vi "ModifyExistingBins.vi"(8 "error in (no error)":errorcluster, 11 "Node Ptr":u64 format="%.0x") -> (0 "error out":errorcluster)   [LabVIEW 2012, in "Histogram Custom Device.lvlib"]
uses:
  Histogram Custom Device.lvlib
  BinBounds.ctl
  <vilib>/NI Veristand/Custom Device API/Custom Device API.lvlib
  <vilib>/NI Veristand/Custom Device API/Get Item Property (Variant).vi
  <vilib>/NI Veristand/Custom Device API/Custom Device Channel Type.ctl
panel:
  in  "Tag":string
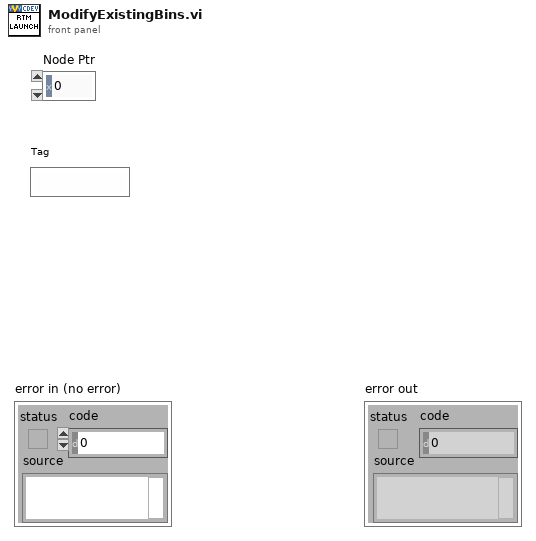
[diagram p1: front panel]
types:
  T1 = typedef "Histogram Custom Device.lvlib/BinBounds.ctl" = cluster{"Bin Counts":i32[], "Upper Bounds":dbl[], "Lower Bounds":dbl[]}
  T2 = typedef "Custom Device API.lvlib/Custom Device Channel Type.ctl" = enum16{"Input", "Output"}
  T3 = typedef "Custom Device API.lvlib/Custom Device Item Ref.ctl" = u64
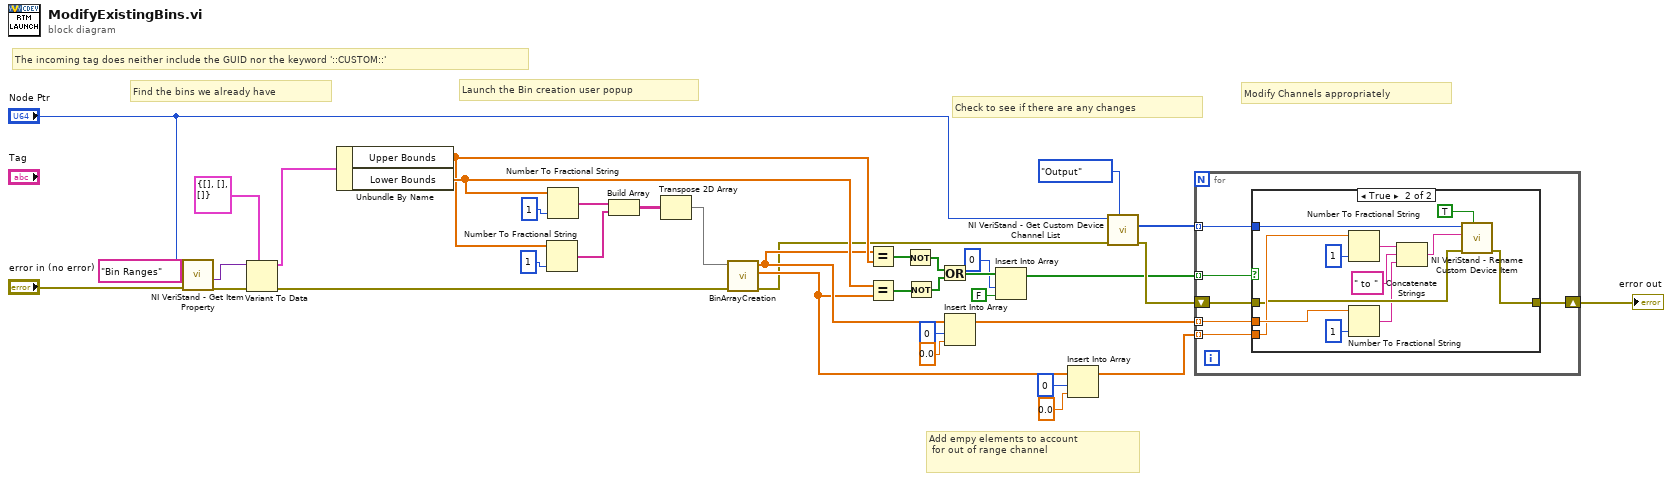
[diagram p0: block diagram]
diagram:
  # "Add empy elements to account\n for out of range channel"
  # "Modify Channels appropriately"
  # "Check to see if there are any changes"
  # "Launch the Bin creation user popup"
  # "Find the bins we already have"
  # "The incoming tag does neither include the GUID nor the keyword '::CUSTOM::'"
  n1 = call-poly <vilib>:"NI VeriStand - Get Item Property.vi"("error in (no error)"="error in (no error)", "Property Name"="Bin Ranges", "Item Ref in"="Node Ptr") -> ("error out"=w8:errorcluster, "Value"=w7:variant)  [unwired: 5 in, 2 out]
  n2 = Variant To Data(error in=w8, type=T1 {"Bin Counts"=[], "Upper Bounds"=[], "Lower Bounds"=[]} ("Cluster"), Variant=w7) -> (data=w20:T1, error out=w2:errorcluster)
  n3 = Unbundle By Name(w20) -> ("Upper Bounds"=w11:dbl[], "Lower Bounds"=w12:dbl[])
  n4 = Number To Fractional String(number=w11, precision (6)=i16 1) -> (F-format string=w16:string[])  [unwired: 2 in]
  n5 = Number To Fractional String(number=w12, precision (6)=i16 1) -> (F-format string=w15:string[])  [unwired: 2 in]
  n6 = Build Array(w15, w16) -> (w10:string[][])
  n7 = Transpose 2D Array(2D array=w10) -> (transposed array=w5:string[][])
  n8 = call "BinArrayCreation.vi"("error in (no error)"=w2, "Histogram Bins"=w5) -> ("error out"=w1:errorcluster, "Lower Bounds"=w3:dbl[], "Upper Bounds"=w4:dbl[])  [unwired: 7 in]
  n9 = Equal?(x=w4, y=w11) -> (x = y?=w26:bool[])
  n10 = Equal?(x=w12, y=w3) -> (x = y?=w27:bool[])
  n11 = Not(x=w26) -> (.not. x?=w25:bool[])
  n12 = Not(x=w27) -> (.not. x?=w24:bool[])
  n13 = Or(x=w25, y=w24) -> (x .or. y?=w23:bool[])
  n14 = Insert Into Array(array=w4, index=0, new element=0.0 ("new element/subarray")) -> (w35:dbl[])
  n15 = Insert Into Array(array=w23, index=0, new element=FALSE ("new element/subarray")) -> (w29:bool[])
  n16 = Insert Into Array(array=w3, index=0, new element=0.0 ("new element/subarray")) -> (w32:dbl[])
  n17 = call <vilib>:"NI VeriStand - Get Custom Device Channel List.vi"("Channel Type"=Custom_Device_Channel_Type."Output", "error in (no error)"=w1, "Device Ref in"="Node Ptr") -> ("error out"=w30:errorcluster, "Specified Channel Ref List"=w28:T3[])  [unwired: 6 in, 1 out]
  n18 = for {
    tunnel: w28 -> [w42] mode=indexing
    tunnel: w29 -> [w43] mode=indexing
    tunnel: w32 -> [w40] mode=indexing
    tunnel: w35 -> [w41] mode=indexing
    shift-right: [w38] -> w17
    shift-left: w30 -> [w39]
    n19 = case shown="True" w43 {
      tunnel: w42 -> [_ w56]
      tunnel: w41 -> [_ w54]
      tunnel: w40 -> [_ w53]
      tunnel: w39 -> [w44 w52]
      tunnel: [w44 w51] -> w38
      frame False {
        # "Do nothing"
      }
      frame True {
        n20 = Number To Fractional String(number=w53, precision (6)=i16 1) -> (F-format string=w45:string)  [unwired: 2 in]
        n21 = Number To Fractional String(number=w54, precision (6)=i16 1) -> (F-format string=w46:string)  [unwired: 2 in]
        n22 = Concatenate Strings(w45, " to " ("string"), w46) -> (w55:string)
        n23 = call <vilib>:"NI VeriStand - Rename Custom Device Item.vi"("Force Rename (F)"=TRUE, "error in (no error)"=w52, "New Name"=w55, "Item Ref in"=w56) -> ("error out"=w51:errorcluster)  [unwired: 5 in, 2 out]
      }
    }
  }
  "error out" <- w17
